vi "Launch Nested Models.vi"(8 "error in (no error)":errorcluster, 10 "Nested Models":refnum<class "IModel.lvclass">[](array[class]), 11 "IModel in":refnum<class "IModel.lvclass">) -> (0 "error out":errorcluster, 3 "IModel out":refnum<class "IModel.lvclass">)   [LabVIEW 2015, in "IModel.lvlib" / "IModel.lvclass"]
uses:
  IModel.lvclass
  IModel.lvclass/IModel.ctl
  <vilib>/ActorFramework/Actor/Actor.lvclass
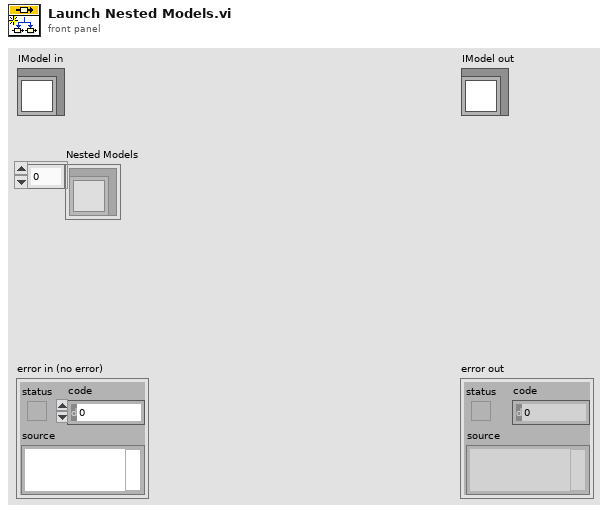
[diagram p1: front panel]
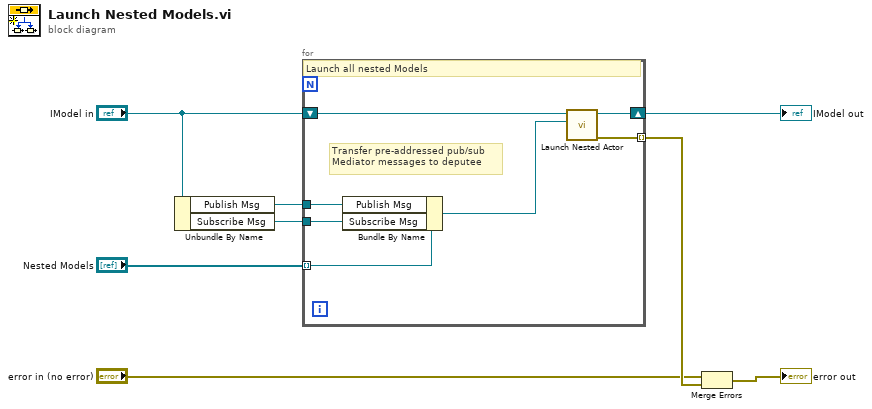
[diagram p0: block diagram]
diagram:
  n1 = Unbundle By Name("IModel in") -> ("Publish Msg"=w2:refnum<class "Publish Msg.lvclass">, "Subscribe Msg"=w1:refnum<class "Subscribe Msg.lvclass">)
  n2 = for {
    shift-right: [w14] -> w8
    shift-left: "IModel in" -> [w15]
    tunnel: "Nested Models" -> [w13] mode=indexing
    tunnel: [w12] -> w6 mode=indexing
    tunnel: w2 -> [w10]
    tunnel: w1 -> [w9]
    # "Transfer pre-addressed pub/sub\nMediator messages to deputee"
    # "Launch all nested Models"
    n3 = Bundle By Name(cluster=w13, "Publish Msg"=w10, "Subscribe Msg"=w9) -> (w11:refnum<class "IModel.lvclass">)
    n4 = call <vilib>:"Launch Nested Actor.vi"("Nested Actor"=w11, "Caller Actor in"=w15) -> ("error out"=w12:errorcluster, "Caller Actor out"=w14:refnum<class "IModel.lvclass">)  [unwired: 7 in, 1 out]
  }
  "IModel out" <- w8
  n5 = Merge Errors("error in (no error)", w6) -> (→"error out":errorcluster)
